vi "TimeShiftDataPoly.vi"   [LabVIEW 2022 SP3]
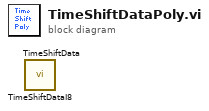
[diagram p0: block diagram]
diagram:
  n1 = call "TimeShiftDataI8.vi"() -> ()  [unwired: 3 in, 2 out]
  n2 = call "TimeShiftData.vi"() -> ()  [unwired: 4 in, 1 out]
